vi "Generate Config Files.vi"(8 "error in":errorcluster, 11 "destination directory":path) -> (0 "error out":errorcluster)   [LabVIEW 2020, in "Template Tool.lvlib"]
uses:
  Template Tool.lvlib
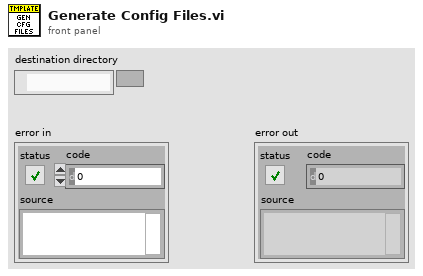
[diagram p1: front panel]
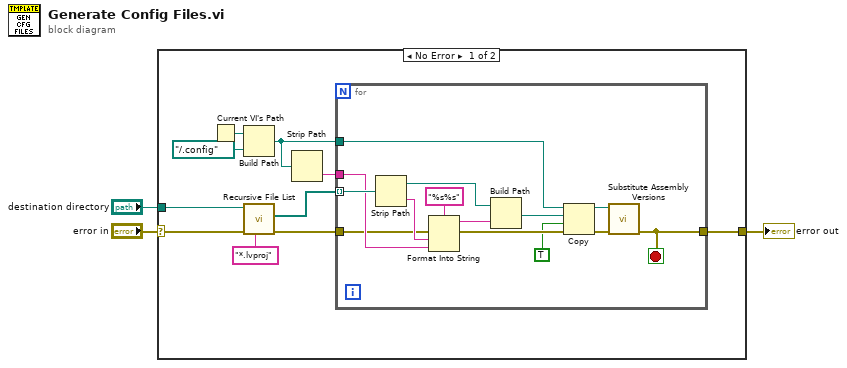
[diagram p0: block diagram]
diagram:
  n1 = case shown="No Error" "error in" {
    selector: "error in" -> [w7 w28]
    tunnel: "destination directory" -> [w5 _]
    tunnel: [w4 w28] -> w1
    frame No Error {
      n2 = Current VI's Path() -> (path=w12:path)
      n3 = Build Path(base path=w12, name or relative path=path "../.config") -> (appended path=w8:path)
      n4 = call <vilib>:"Recursive File List.vi"("pattern"="*.lvproj", "error in (no error)"=w7, "Folder Path"=w5) -> ("error out"=w6:errorcluster, "All Files in Dir"=w10:path[])  [unwired: 4 in, 3 out]
      n5 = Strip Path(path=w8) -> (name=w9:string)  [unwired: 1 out]
      n6 = for {
        tunnel: w10 -> [w27] mode=indexing
        tunnel: w9 -> [w24]
        tunnel: w8 -> [w20]
        tunnel: w6 -> [w19]
        tunnel: [w14] -> w4
        stop <- w14 stop-if-true
        n7 = Strip Path(path=w27) -> (stripped path=w23:path, name=w25:string)
        n8 = Format Into String(format string="%s%s", error in=w19, w25, w24) -> (resulting string=w22:string, error out=w18:errorcluster)  [unwired: 1 in]
        n9 = Build Path(base path=w23, name or relative path=w22) -> (appended path=w21:path)
        n10 = Copy(8:w18, 9:TRUE ("overwrite (F)"), 10:w21, 11:w20) -> (0:w16:errorcluster, 3:w15:path)  [unwired: 1 in, 1 out]
        n11 = call "Substitute Assembly Versions.vi"("error in"=w16, "config file path"=w15) -> ("error out"=w14:errorcluster)  [unwired: 9 in]
      }
    }
    frame Error {
    }
  }
  "error out" <- w1
